vi "Init Close eFGV.vi"(6 "State - eFGV":T1=enum."Close", 8 "error in (no error)":errorcluster) -> (0 "error out":errorcluster)   [LabVIEW 2020]
uses:
  Control/State - eFGV.ctl
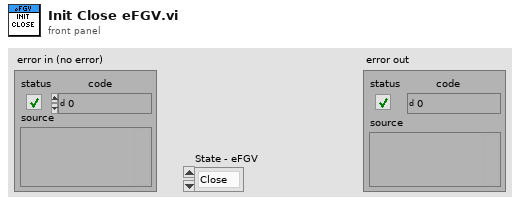
[diagram p1: front panel]
types:
  T1 = typedef "State - eFGV.ctl" = enum16{"Init", "Read", "Write", "Close"}
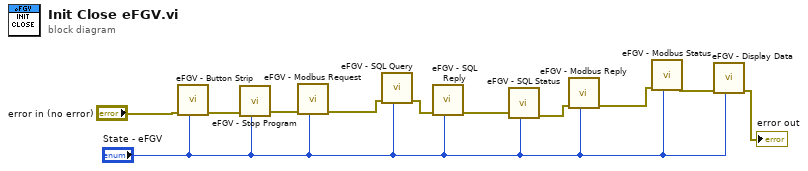
[diagram p0: block diagram]
diagram:
  n1 = call "eFGV - Button Strip.vi"("State - eFGV"="State - eFGV", "error in (no error)"="error in (no error)") -> ("error out"=w10:errorcluster)  [unwired: 8 in, 1 out]
  n2 = call "eFGV - Stop Program.vi"("State - eFGV"="State - eFGV", "error in (no error)"=w10) -> ("error out"=w9:errorcluster)  [unwired: 8 in, 1 out]
  n3 = call "eFGV - Modbus Request.vi"("State - eFGV"="State - eFGV", "error in (no error)"=w9) -> ("error out"=w8:errorcluster)  [unwired: 8 in, 1 out]
  n4 = call "eFGV - SQL Query.vi"("State"="State - eFGV", "error in (no error)"=w8) -> ("error out"=w7:errorcluster)  [unwired: 8 in, 1 out]
  n5 = call "eFGV - SQL Reply.vi"("State"="State - eFGV", "error in (no error)"=w7) -> ("error out"=w6:errorcluster)  [unwired: 8 in, 1 out]
  n6 = call "eFGV - SQL Status.vi"("State"="State - eFGV", "error in (no error)"=w6) -> ("error out"=w5:errorcluster)  [unwired: 8 in, 1 out]
  n7 = call "eFGV - Modbus Reply.vi"("State - eFGV"="State - eFGV", "error in (no error)"=w5) -> ("error out"=w4:errorcluster)  [unwired: 8 in, 1 out]
  n8 = call "eFGV - Modbus Status.vi"("State - eFGV"="State - eFGV", "error in (no error)"=w4) -> ("error out"=w3:errorcluster)  [unwired: 8 in, 1 out]
  n9 = call "eFGV - Display Data.vi"("State - eFGV"="State - eFGV", "error in (no error)"=w3) -> ("error out"=→"error out":errorcluster)  [unwired: 8 in, 1 out]
